vi "Generate Key Accept.vi"(11 "Sec-WebSocket-Key":string="dGhlIHNhbXBsZSBub25jZQ==") -> (3 "Sec-WebSocket-Accept":string)   [LabVIEW 2020, in "Stream-Websocket.lvlib"]
uses:
  Stream-Websocket.lvlib
  <vilib>/IlluminatedG/lv-web-crypto/lv-crypto/Crypto/SHA-1/SHA-1.lvclass
  <vilib>/IlluminatedG/lv-web-crypto/lv-base64/Base64.lvlib
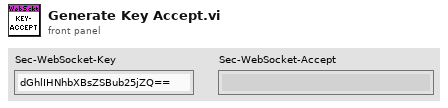
[diagram p1: front panel]
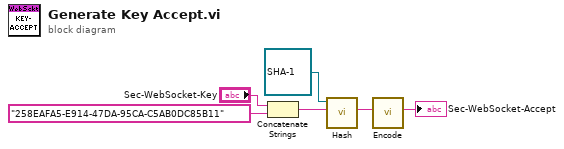
[diagram p0: block diagram]
diagram:
  n1 = Concatenate Strings("Sec-WebSocket-Key", "258EAFA5-E914-47DA-95CA-C5AB0DC85B11") -> (w4:string)
  n2 = call-dynamic "Hash.vi"("Message"=w4, "SHA-1 in"=refnum<class "SHA-1.lvclass"> refnum) -> ("Hash"=w2:string)  [unwired: 7 in, 2 out]
  n3 = call <vilib>:"Encode.vi"("string in (not encoded)"=w2) -> ("string out (base64-encoded)"=→"Sec-WebSocket-Accept":string)  [unwired: 9 in, 1 out]
